vi "Configuration File PAth -- Constant.vi"() -> (3 "Configuration File Path":path)   [LabVIEW 2018]
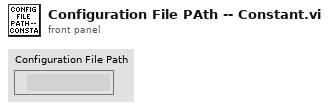
[diagram p1: front panel]
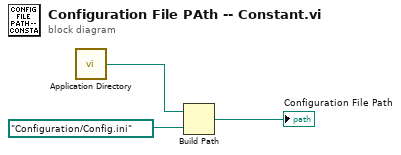
[diagram p0: block diagram]
diagram:
  n1 = call <vilib>:"Application Directory.vi"() -> ("Application Directory"=w2:path)
  n2 = Build Path(base path=w2, name or relative path=path "Configuration/Config.ini") -> (appended path=→"Configuration File Path":path)
